vi "get data.vi"(7 "Board number":i32, 8 "error in (no error)":errorcluster, 11 "Measurement config":T1={"Range"=3, "Rate (Hz)"=1200000, "Count"=480000, "HighChan"=3, "LowChan"=0} {"Range" items=["Not Programmable"=0, "+- 20 V"=27, "+- 10 V"=1, "+- 5 V"=2, "+- 4 V"=28, "+- 2.5 V"=3, "+- 2 V"=29, "+- 1.67 V"=4, "+- 1.25 V"=5, "+- 1 V"=6, "+- .625 V"=7, "+- .5 V"=8, "+- .25 V"=30, "+- .2 V"=31, "+- .1 V"=9, "+- .05 V"=10, "+- .01 V"=11, "+- .005 V"=12, "0 - 10 V"=13, "0 - 5 V"=14, "0 - 4 V"=36, "0 - 2.5 V"=15, "0 - 2 V"=16, "0 - 1.67 V"=17, "0 - 1.25 V"=18, "0 - 1 V"=19, "0 - .5 V"=32, "0 - .25 V"=33, "0 - .2 V"=34, "0 - .1 V"=20, "0 - .02 V"=35, "0 - .01 V"=21, "4 - 20 mA"=22, "2 - 10 mA"=23, "1 - 5 mA"=24, ".5 - 2.5 mA"=25, "0 - 20 mA"=26]}) -> (0 "error out":errorcluster, 1 "Start time":timestamp, 2 "Data":sgl[](array[numeric]) format="%.2f", 3 "Measurement config out":T1={"Range"=3, "Rate (Hz)"=1200000, "Count"=480000, "HighChan"=3, "LowChan"=0} {"Range" items=["Not Programmable"=0, "+- 20 V"=27, "+- 10 V"=1, "+- 5 V"=2, "+- 4 V"=28, "+- 2.5 V"=3, "+- 2 V"=29, "+- 1.67 V"=4, "+- 1.25 V"=5, "+- 1 V"=6, "+- .625 V"=7, "+- .5 V"=8, "+- .25 V"=30, "+- .2 V"=31, "+- .1 V"=9, "+- .05 V"=10, "+- .01 V"=11, "+- .005 V"=12, "0 - 10 V"=13, "0 - 5 V"=14, "0 - 4 V"=36, "0 - 2.5 V"=15, "0 - 2 V"=16, "0 - 1.67 V"=17, "0 - 1.25 V"=18, "0 - 1 V"=19, "0 - .5 V"=32, "0 - .25 V"=33, "0 - .2 V"=34, "0 - .1 V"=20, "0 - .02 V"=35, "0 - .01 V"=21, "4 - 20 mA"=22, "2 - 10 mA"=23, "1 - 5 mA"=24, ".5 - 2.5 mA"=25, "0 - 20 mA"=26]})   [LabVIEW 2019, in "DAQ_Engine.lvclass"]
doc: "Developed by Kevin Thompson\nkevin@thompsonengineering.net\n\nCopyright 2020\nThompson Engineering, LLC"
uses:
  DAQ_Engine.lvclass
  ToEng(array).vi
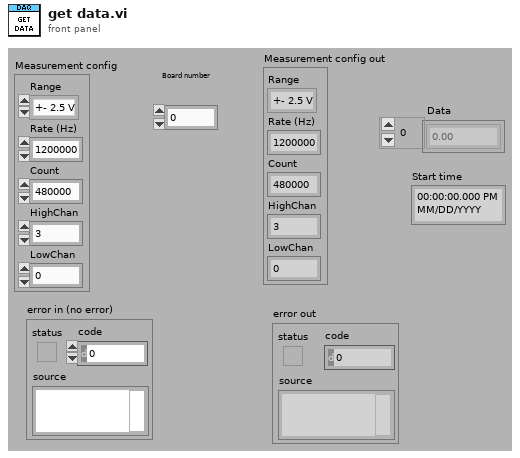
[diagram p1: front panel]
types:
  T1 = cluster{"Range":i32, "Rate (Hz)":i32, "Count":i32, "HighChan":i32, "LowChan":i32}
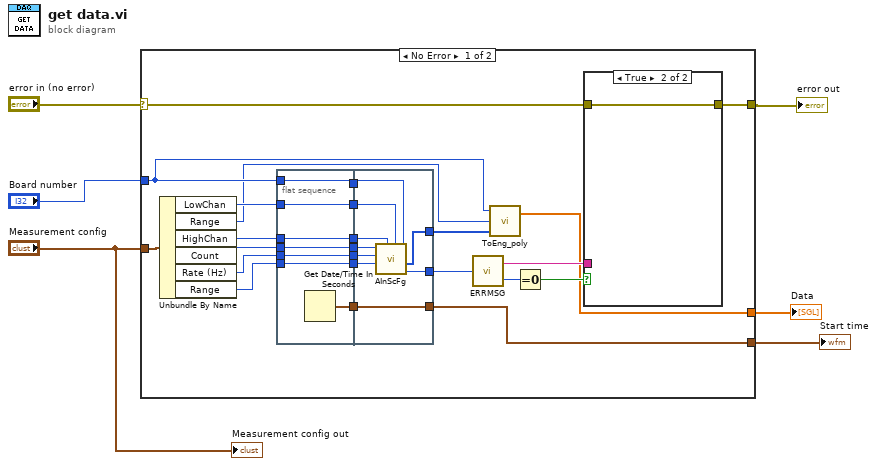
[diagram p0: block diagram]
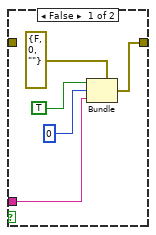
[diagram p2: hidden frame]
diagram:
  n1 = case shown="No Error" "error in (no error)" {
    selector: "error in (no error)" -> [w21 w53]
    tunnel: [w20 w53] -> w6
    tunnel: "Board number" -> [w18 _]
    tunnel: "Measurement config" -> [w28 _]
    tunnel: [w8 _] -> w1
    tunnel: [w7 _] -> w2
    frame No Error {
      n2 = Unbundle By Name(w28) -> ("LowChan"=w26:i32, "Range"=w17:i32, "HighChan"=w27:i32, "Count"=w25:i32, "Rate (Hz)"=w24:i32, "Range"=w23:i32)
      n3 = flat-sequence {
        tunnel: w18 -> [w32]
        tunnel: w23 -> [w33]
        tunnel: w24 -> [w34]
        tunnel: w25 -> [w35]
        tunnel: w26 -> [w36]
        tunnel: w27 -> [w37]
        tunnel: [w37] -> w15
        tunnel: [w36] -> w14
        tunnel: [w35] -> w13
        tunnel: [w34] -> w12
        tunnel: [w33] -> w11
        tunnel: [w32] -> w10
        tunnel: [w31] -> w9
        tunnel: [w46] -> w30
        tunnel: [w39] -> w16
        tunnel: w15 -> [w45]
        tunnel: w14 -> [w44]
        tunnel: w13 -> [w43]
        tunnel: w12 -> [w42]
        tunnel: w11 -> [w41]
        tunnel: w10 -> [w40]
        tunnel: [w38] -> w8
        tunnel: w9 -> [w38]
        frame #0 {
          n4 = Get Date/Time In Seconds() -> (seconds since 1Jan1904=w31:timestamp)
        }
        frame #1 {
          n5 = call "AInScFg.VI"("BoardNum"=w40, "LowChan"=w44, "HighChan"=w45, "Range"=w41, "Rate"=w42, "Count"=w43) -> ("ErrCode"=w46:i32, "ADData"=w39:u16[])  [unwired: 2 in, 1 out]
        }
      }
      n6 = call "ERRMSG.VI"("ErrCode"=w30) -> ("ErrMsg"=w19:string, "ErrCode (Out)"=w29:i32)
      n7 = call-poly "ToEng_poly.VI"("AD Data"=w16, "Range"=w17, "BoardNum"=w18) -> ("Eng Units"=w7:sgl[])  [unwired: 1 out]
      n8 = Equal To 0?(x=w29) -> (x = 0?=w22:bool)
      n9 = case shown="True" w22 {
        tunnel: w21 -> [_ w52]
        tunnel: [w50 w52] -> w20
        tunnel: w19 -> [w48 _]
        frame False {
          n10 = Bundle(cluster=errorcluster {"status"=FALSE, "code"=0, "source"=""} ("error IO"), "status"=TRUE, "code"=0, "source"=w48) -> (w50:errorcluster)
        }
        frame True {
        }
      }
    }
    frame Error {
    }
  }
  "error out" <- w6
  "Data" <- w2
  "Start time" <- w1
  "Measurement config out" <- "Measurement config"
